vi "sub_main_ledmatrix.vi"(8 "error in":errorcluster) -> (0 "error out":errorcluster)   [LabVIEW 2019]
uses:
  Ctrl/cmd_common.ctl
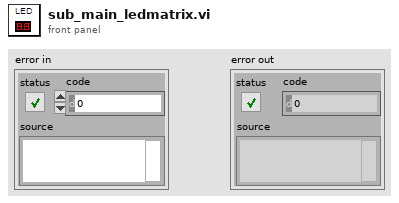
[diagram p1: front panel]
types:
  T1 = typedef "cmd_common.ctl" = enum16{"read", "write"}
  T2 = typedef "error_cluster.ctl" = cluster{"AGV":u8, "AGV Estop":u8, "Obstacle":u8, "Heading":u8, "Waypt":u8, "GNSS":u8, "VLP16":u8, "Cam":u8, "RPLidar":u8, "Joystick":u8, "IMU":u8, "Led":u8}
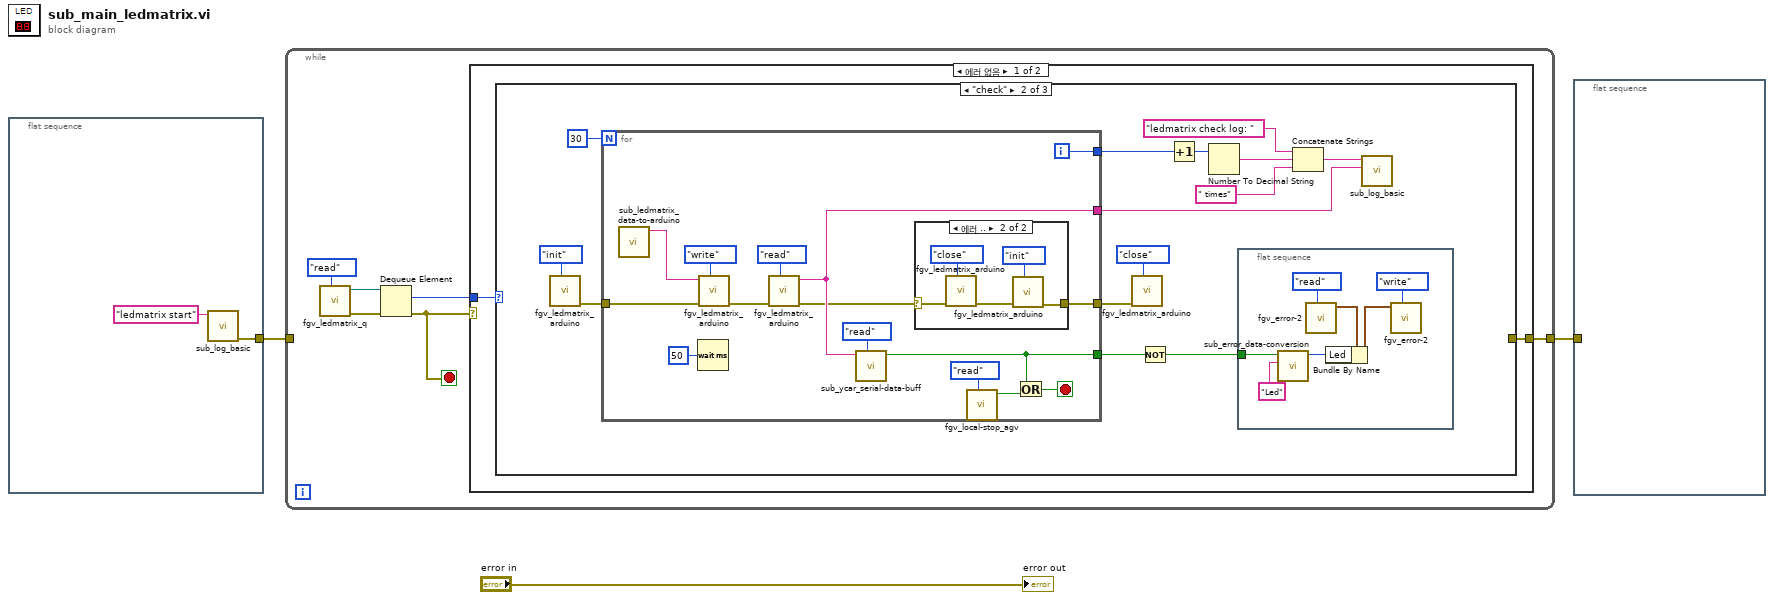
[diagram p0: block diagram]
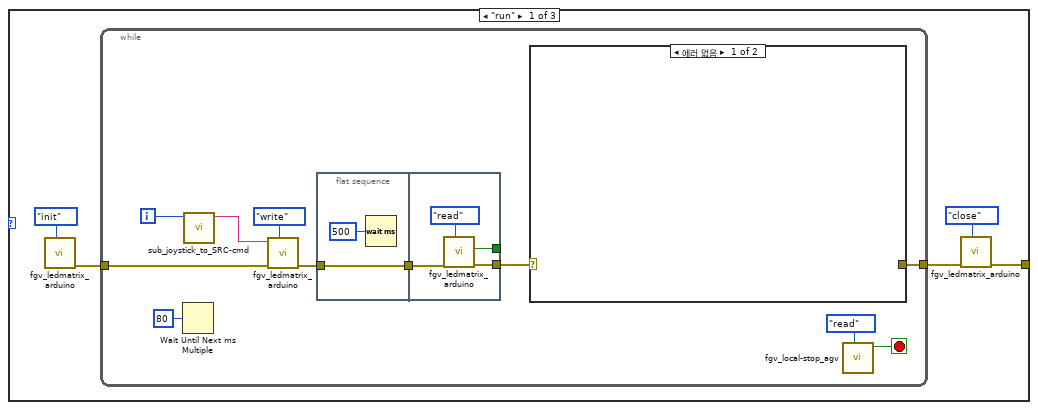
[diagram p2: hidden frame]
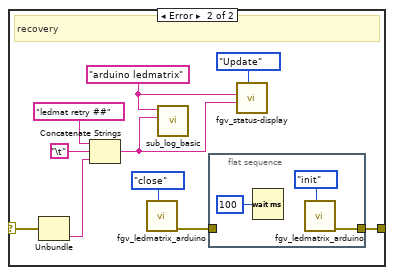
[diagram p3: hidden frame]
diagram:
  n1 = flat-sequence {
    tunnel: [w4] -> w1
    frame #0 {
      n2 = call "sub_log_basic.vi"("Title"="ledmatrix start") -> ("error out"=w4:errorcluster)  [unwired: 10 in]
    }
  }
  n3 = while {
    tunnel: [w7] -> w3
    tunnel: w1 -> [_]
    stop <- w6 stop-if-true
    n4 = call "fgv_ledmatrix_q.vi"("cmd"=enum16{"create", "write", "read", "close"}."read") -> ("error out"=w10:errorcluster, "queue out"=w9:refnum<queue>)  [unwired: 9 in]
    n5 = Dequeue Element(queue=w9, error in (no error)=w10) -> (element=w8:enum16{"run", "check", "stop"}, error out=w6:errorcluster)  [unwired: 1 in, 2 out]
    n6 = case shown="에러 없음" w6 {
      tunnel: w8 -> [w13 _]
      tunnel: [w12 _] -> w7
      frame No Error {
        n7 = case shown="\"check\"" w13 {
          tunnel: [w14 _ _] -> w12
          frame "run" {
            n8 = call "fgv_ledmatrix_arduino.vi"("cmd"=enum16{"init", "read", "write", "close"}."init") -> ("error out"=w16:errorcluster)  [unwired: 8 in, 2 out]
            n9 = while {
              tunnel: w16 -> [w25]
              tunnel: [w22] -> w15
              i -> [w19]
              stop <- w28 stop-if-true
              n10 = Wait Until Next ms Multiple(millisecond multiple=u32 80 ("milliseconds to wait")) -> ()  [unwired: 1 out]
              n11 = call "sub_joystick_to_SRC-cmd.vi"("index"=w19) -> ("cmd out"=w20:string)  [unwired: 9 in, 1 out]
              n12 = call "fgv_ledmatrix_arduino.vi"("cmd"=enum16{"init", "read", "write", "close"}."write", "error in"=w25, "cmd 2"=w20) -> ("error out"=w26:errorcluster)  [unwired: 6 in, 2 out]
              n13 = flat-sequence {
                tunnel: w26 -> [w44]
                tunnel: [w44] -> w23
                tunnel: [w46] -> w21
                tunnel: w23 -> [w47]
                tunnel: [w45] -> _
                frame #0 {
                  n14 = Wait (ms)(milliseconds to wait=u32 500) -> ()  [unwired: 1 out]
                }
                frame #1 {
                  n15 = call "fgv_ledmatrix_arduino.vi"("cmd"=enum16{"init", "read", "write", "close"}."read", "error in"=w47) -> ("error out"=w46:errorcluster, "val"=w45:bool)  [unwired: 7 in, 1 out]
                }
              }
              n16 = case shown="에러 없음" w21 {
                selector: w21 -> [_ w34]
                tunnel: [_ w37] -> w22
                frame No Error {
                }
                frame Error {
                  w35 = "arduino ledmatrix" ("Title")
                  # "recovery"
                  n17 = Unbundle(w34) -> ("source"=w31:string)  [unwired: 2 out]
                  n18 = Concatenate Strings("ledmat retry ##" ("desc"), "\t", w31) -> (w32:string)
                  n19 = call "fgv_ledmatrix_arduino.vi"("cmd"=enum16{"init", "read", "write", "close"}."close") -> ("error out"=w38:errorcluster)  [unwired: 8 in, 2 out]
                  n20 = call "sub_log_basic.vi"("desc"=w32, "Title"=w35) -> ()  [unwired: 9 in, 1 out]
                  n21 = flat-sequence {
                    tunnel: w38 -> [_]
                    tunnel: [w41] -> w37
                    frame #0 {
                      n22 = Wait (ms)(milliseconds to wait=u32 100) -> ()  [unwired: 1 out]
                      n23 = call "fgv_ledmatrix_arduino.vi"("cmd"=enum16{"init", "read", "write", "close"}."init") -> ("error out"=w41:errorcluster)  [unwired: 8 in, 2 out]
                    }
                  }
                  n24 = call "fgv_status-display.vi"("Mode"=enum16{"Initial", "Update", "Clear"}."Update", "detail"=w32, "title"=w35) -> ()  [unwired: 8 in, 1 out]
                }
              }
              n25 = call "fgv_local-stop_agv.vi"("cmd"=enum16{"ini", "read", "stop"}."read") -> ("stop status"=w28:bool)  [unwired: 10 in]
            }
            n26 = call "fgv_ledmatrix_arduino.vi"("cmd"=enum16{"init", "read", "write", "close"}."close", "error in"=w15) -> ("error out"=w14:errorcluster)  [unwired: 7 in, 2 out]
          }
          frame "check" {
            n27 = call "fgv_ledmatrix_arduino.vi"("cmd"=enum16{"init", "read", "write", "close"}."init") -> ("error out"=w50:errorcluster)  [unwired: 8 in, 2 out]
            n28 = for {
              N: 30 -> [_]
              tunnel: [w80] -> w53
              tunnel: [w77] -> w52
              tunnel: [w76] -> w51
              tunnel: w50 -> [w73]
              tunnel: [w71] -> w49
              i -> [w80]
              stop <- w79 stop-if-true
              n29 = call "sub_ledmatrix_data-to-arduino.vi"() -> ("data out"=w70:string)  [unwired: 10 in, 1 out]
              n30 = Wait (ms)(milliseconds to wait=u32 50) -> ()  [unwired: 1 out]
              n31 = call "fgv_ledmatrix_arduino.vi"("cmd"=enum16{"init", "read", "write", "close"}."write", "error in"=w73, "cmd 2"=w70) -> ("error out"=w81:errorcluster)  [unwired: 6 in, 2 out]
              n32 = call "fgv_ledmatrix_arduino.vi"("cmd"=enum16{"init", "read", "write", "close"}."read", "error in"=w81) -> ("error out"=w72:errorcluster, "read_buffer"=w77:string)  [unwired: 7 in, 1 out]
              n33 = call "sub_ycar_serial-data-buff.vi"("cmd"=cmd_common."read", "data"=w77) -> ("val"=w76:bool)  [unwired: 8 in, 1 out]
              n34 = case shown="에러 .." w72 {
                selector: w72 -> [w85 w89]
                tunnel: [w85 w87] -> w71
                frame No Error {
                }
                frame Error {
                  n35 = call "fgv_ledmatrix_arduino.vi"("cmd"=enum16{"init", "read", "write", "close"}."close", "error in"=w89) -> ("error out"=w86:errorcluster)  [unwired: 7 in, 2 out]
                  n36 = call "fgv_ledmatrix_arduino.vi"("cmd"=enum16{"init", "read", "write", "close"}."init", "error in"=w86) -> ("error out"=w87:errorcluster)  [unwired: 7 in, 2 out]
                }
              }
              n37 = call "fgv_local-stop_agv.vi"("cmd"=enum16{"ini", "read", "stop"}."read") -> ("stop status"=w74:bool)  [unwired: 10 in]
              n38 = Or(x=w76, y=w74) -> (x .or. y?=w79:bool)
            }
            n39 = call "fgv_ledmatrix_arduino.vi"("cmd"=enum16{"init", "read", "write", "close"}."close", "error in"=w49) -> ()  [unwired: 7 in, 3 out]
            n40 = Not(x=w51) -> (.not. x?=w59:bool)
            n41 = Increment(x=w53) -> (x+1=w56:i32)
            n42 = Number To Decimal String(number=w56) -> (decimal integer string=w57:string)  [unwired: 1 in]
            n43 = flat-sequence {
              tunnel: w59 -> [w64]
              frame #0 {
                n44 = call "sub_error_data-conversion.vi"("name"="Led", "error status"=w64) -> ("error conversion out"=w69:u8)  [unwired: 8 in, 1 out]
                n45 = call "fgv_error-2.vi"("cmd"=enum16{"init", "read", "write"}."read") -> ("Error cluster out"=w68:T2)  [unwired: 9 in, 1 out]
                n46 = Bundle By Name(cluster=w68, "Led"=w69) -> (w67:T2)
                n47 = call "fgv_error-2.vi"("cmd"=enum16{"init", "read", "write"}."write", "Error cluster"=w67) -> ()  [unwired: 8 in, 2 out]
              }
            }
            n48 = Concatenate Strings("ledmatrix check log: " ("Title"), w57, " times" ("문자열")) -> (w58:string)
            n49 = call "sub_log_basic.vi"("desc"=w52, "Title"=w58) -> ()  [unwired: 9 in, 1 out]
          }
          frame "stop", Default {
          }
        }
      }
      frame Error {
      }
    }
  }
  n50 = flat-sequence {
    tunnel: w3 -> [_]
    frame #0 {
    }
  }
  "error out" <- "error in"
